vi "TUNA parse the data.vi"(0 "Nav String":string="$,G,43,13,230,P,10,20,120,T,10,10,330,L,14,36,110,A,3,5,B,7,8,C,16,20,D,-1,-1,S,08,12,234\r", 1 "Tug":string="G") -> (2 "Buoy locations":cluster{"regular expression":string, i32, i32}[](array[cluster]), 3 "Tug Location":T1, 4 "Time":cluster{i32, i32, i32}, 5 "Valid?":bool)   [LabVIEW 2014]
doc: "This VI find the position of the tug whose letter was passed: X, Y and Heading.. The position values are positions are in pixel locations with 0,0 being at the top left, the heading is in degrees. It also finds the buoy locations and the time in hrs, min , secs."
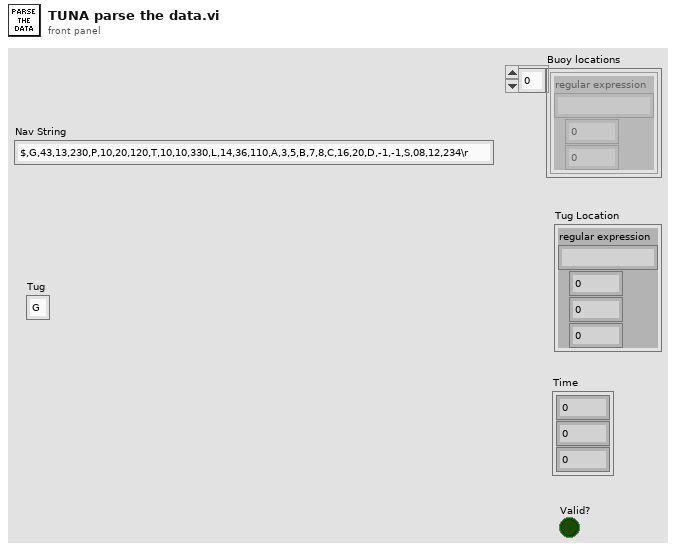
[diagram p1: front panel]
types:
  T1 = cluster{"regular expression":string, i32, i32, i32}
  T2 = cluster{"X POS":i32, "Y POS":i32, "HEADING":dbl}[]
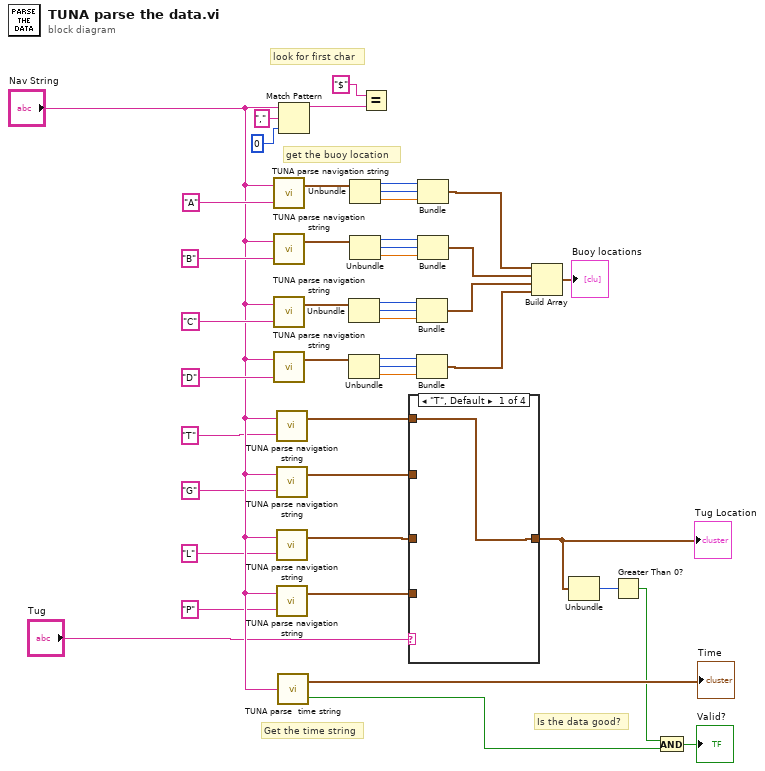
[diagram p0: block diagram]
diagram:
  # "Is the data good?"
  # "get the buoy location"
  # "Get the time string"
  # "look for first char"
  n1 = call "TUNA parse navigation string.vi"("Header"="A" ("Tug"), "Nav String"="Nav String") -> ("Output GPS"=w40:cluster{"X POS":i32, "Y POS":i32, "HEADING":dbl})  [unwired: 1 out]
  n2 = call "TUNA parse navigation string.vi"("Header"="B" ("Tug"), "Nav String"="Nav String") -> ("Output GPS"=w35:cluster{"X POS":i32, "Y POS":i32, "HEADING":dbl})  [unwired: 1 out]
  n3 = call "TUNA parse navigation string.vi"("Header"="C" ("Tug"), "Nav String"="Nav String") -> ("Output GPS"=w30:cluster{"X POS":i32, "Y POS":i32, "HEADING":dbl})  [unwired: 1 out]
  n4 = call "TUNA parse navigation string.vi"("Header"="D" ("Tug"), "Nav String"="Nav String") -> ("Output GPS"=w25:cluster{"X POS":i32, "Y POS":i32, "HEADING":dbl})  [unwired: 1 out]
  n5 = call "TUNA parse navigation string.vi"("Header"="T", "Nav String"="Nav String") -> ("Output GPS"=w10:cluster{"X POS":i32, "Y POS":i32, "HEADING":dbl})  [unwired: 1 out]
  n6 = call "TUNA parse navigation string.vi"("Header"="G", "Nav String"="Nav String") -> ("Output GPS"=w9:cluster{"X POS":i32, "Y POS":i32, "HEADING":dbl})  [unwired: 1 out]
  n7 = call "TUNA parse navigation string.vi"("Header"="L", "Nav String"="Nav String") -> ("Output GPS"=w7:cluster{"X POS":i32, "Y POS":i32, "HEADING":dbl})  [unwired: 1 out]
  n8 = call "TUNA parse navigation string.vi"("Header"="P", "Nav String"="Nav String") -> ("Output GPS"=w6:cluster{"X POS":i32, "Y POS":i32, "HEADING":dbl})  [unwired: 1 out]
  n9 = call "TUNA parse  time string.vi"("Nav String"="Nav String") -> ("output cluster"=→"Time":cluster{i32, i32, i32}, "Valid?"=w2:bool)
  n10 = Match Pattern(string="Nav String", regular expression=",", offset (0)=0) -> (before substring=w44:string)  [unwired: 3 out]
  n11 = Unbundle(w30) -> ("X POS"=w29:i32, "Y POS"=w28:i32, "HEADING"=w27:dbl)
  n12 = Unbundle(w25) -> ("X POS"=w24:i32, "Y POS"=w23:i32, "HEADING"=w22:dbl)
  n13 = Unbundle(w40) -> ("X POS"=w39:i32, "Y POS"=w38:i32, "HEADING"=w37:dbl)
  n14 = Unbundle(w35) -> ("X POS"=w34:i32, "Y POS"=w33:i32, "HEADING"=w32:dbl)
  n15 = Equal?(x="$", y=w44) -> ()  [unwired: 1 out]
  n16 = case shown="\"T\", Default" "Tug" {
    tunnel: w10 -> [w46 _ _ _]
    tunnel: w9 -> [_ w47 _ _]
    tunnel: w7 -> [_ _ w48 _]
    tunnel: w6 -> [_ _ _ w49]
    tunnel: [w46 w47 w48 w49] -> w5
    frame "T", Default {
    }
    frame "G" {
    }
    frame "L" {
    }
    frame "P" {
    }
  }
  "Tug Location" <- w5
  n17 = Bundle("X POS"=w29, "Y POS"=w28, "HEADING"=w27) -> (w19:cluster{"X POS":i32, "Y POS":i32, "HEADING":dbl})  [unwired: 1 in]
  n18 = Bundle("X POS"=w24, "Y POS"=w23, "HEADING"=w22) -> (w18:cluster{"X POS":i32, "Y POS":i32, "HEADING":dbl})  [unwired: 1 in]
  n19 = Bundle("X POS"=w39, "Y POS"=w38, "HEADING"=w37) -> (w21:cluster{"X POS":i32, "Y POS":i32, "HEADING":dbl})  [unwired: 1 in]
  n20 = Bundle("X POS"=w34, "Y POS"=w33, "HEADING"=w32) -> (w20:cluster{"X POS":i32, "Y POS":i32, "HEADING":dbl})  [unwired: 1 in]
  n21 = Build Array(w21, w20, w19, w18) -> (→"Buoy locations":T2)
  n22 = Unbundle(w5) -> ("Y POS"=w4:i32)  [unwired: 2 out]
  n23 = Greater Than 0?(x=w4) -> (x > 0?=w1:bool)
  n24 = And(x=w1, y=w2) -> (x .and. y?=→"Valid?":bool)
